vi "DISP_WIND_TRAC_TITL_STAT.vi"(0 "VISA IN":refnum<visa-resource-name>, 1 "Trace":i32, 2 "ON | OFF":bool, 5 "error in":errorcluster, 7 "Window":i32) -> (14 "VISA Out":refnum<visa-resource-name>, 19 "error out":errorcluster)   [LabVIEW 2018, in "PNA-X.lvlib"]
doc: "DISPlay:WINDow<wnum>:TRACe<tnum>TITLe:STATe <bool> \n(Read-Write) Turns display of the Trace Title ON or OFF. When turned OFF, the previous trace title \nreturns. Set a new trace title using DISP:WIND:TRAC:TITL:DATA \nLearn more about Trace Titles \nParameters \n<wnum> Any existing window number. If unspecified, value is set to 1 \n<tnum> Trace number of the specified window. If unspecified, value is set to 1. The \ntrace number displayed in trace status is the trace number of the channel; not \nthe window. Use Display:Cat? to read the window numbers. Use \nDisp:Window:Cat? to read the trace numbers of the specified window. \n<bool> ON (or 1) - turns the title ON. \nOFF (or 0) - turns the title OFF. \nExamples DISP:WIND:TRAC:TITL ON \nDisplay:window2:trace3:title:state off \nQuery Syntax DISPlay:WINDow<wnum>:TRACe<tnum>:TITLe[:STATe]? \n1598\n\nReturn Type Boolean (1 = ON, 0 = OFF) \nDefault ON"
uses:
  PNA-X.lvlib
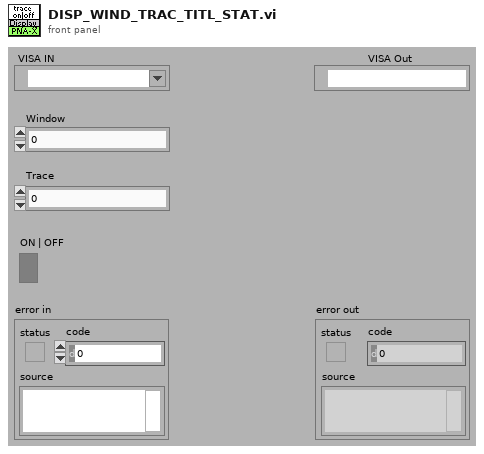
[diagram p1: front panel]
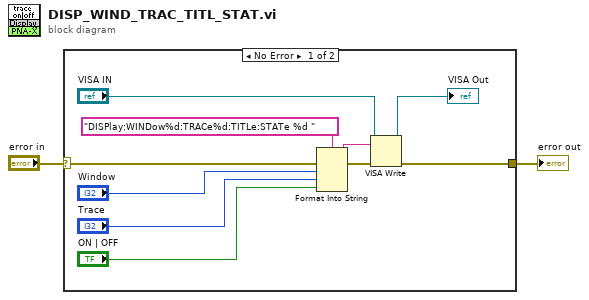
[diagram p0: block diagram]
diagram:
  n1 = case shown="No Error" "error in" {
    selector: "error in" -> [w12 w13]
    tunnel: [w7 w13] -> w1
    frame No Error {
      n2 = Format Into String(format string="DISPlay:WINDow%d:TRACe%d:TITLe:STATe %d " ("Cmdline"), error in=w12, "Window", "Trace", "ON | OFF") -> (resulting string=w10:string, error out=w11:errorcluster)  [unwired: 1 in]
      n3 = VISA Write(VISA resource name="VISA IN", write buffer=w10, error in (no error)=w11) -> (VISA resource name out=→"VISA Out":refnum<visa-resource-name>, error out=w7:errorcluster)  [unwired: 1 out]
    }
    frame Error {
    }
  }
  "error out" <- w1
